vi "FakeTheory.vi"(10 "Input Data":string) -> (0 "error out":errorcluster)   [LabVIEW 2019, in "TestSuiteTestSupport.lvlib"]
uses:
  TestSuiteTestSupport.lvlib
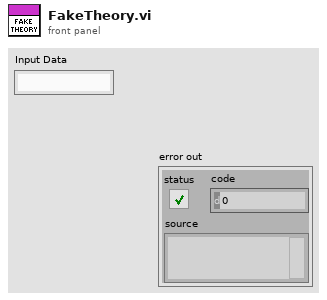
[diagram p1: front panel]
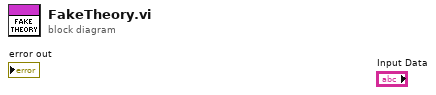
[diagram p0: block diagram]
diagram:
